vi "WPI_DashboardFPS Calculator.vi"(11 "Average Count":i32=30) -> (1 "delta (ms)":u32, 3 "fps":dbl)   [LabVIEW 2017]
doc: "Measure the time between calls and average the last few to smooth the value a bit."
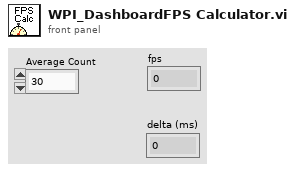
[diagram p1: front panel]
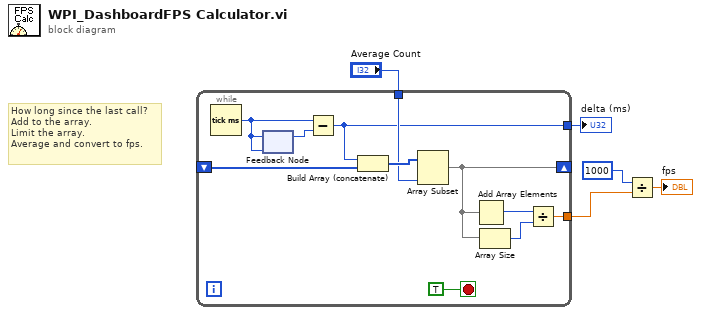
[diagram p0: block diagram]
diagram:
  # "How long since the last call?\nAdd to the array.\nLimit the array.\nAverage and convert to fps."
  n1 = while {
    tunnel: [w13] -> w4
    shift-right: [w7] -> _
    shift-left: _ -> [w12]
    tunnel: "Average Count" -> [w10]
    tunnel: [w6] -> w1
    stop <- TRUE stop-if-true
    n2 = Tick Count (ms)() -> (millisecond timer value=w14:u32)
    n3 = feedback #1(w14) -> (w16:u32)
    n4 = feedback-in #1(w14) -> ()
    n5 = Subtract(x=w14, y=w16) -> (x-y=w6:u32)
    n6 = Build Array (concatenate)(w6, w12) -> (w11:u32[])
    n7 = Array Subset(array=w11, length=w10) -> (w7:u32[])  [unwired: 1 in]
    n8 = Add Array Elements(numeric array=w7) -> (sum=w8:u32)
    n9 = Array Size(array=w7) -> (size(s)=w9:i32)
    n10 = Divide(x=w8, y=w9) -> (x/y=w13:dbl)
  }
  "delta (ms)" <- w1
  n11 = Divide(x=1000, y=w4) -> (x/y=→"fps":dbl)
